vi "GetBounds 1.vi"(0 "XRef":T5, 1 "State In":T4) -> (14 "Bounds":T2, 15 "Fatal Error Out":T1)   [LabVIEW 2012, in "VireoFunctionNode.xnode"]
uses:
  VireoFunctionNode.xnode
  <vilib>/XNodeSupport/XNodeXNodeRef.ctl
  State 1.ctl
  <vilib>/XNodeSupport/XNodeBounds.ctl
  <vilib>/XNodeSupport/XNodeInt.ctl
  <vilib>/XNodeSupport/XNodeErrorCluster.ctl
  <vilib>/XNodeSupport/NI_XNodeSupport.lvlib
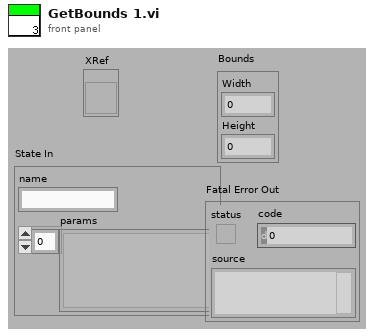
[diagram p1: front panel]
types:
  T1 = typedef "NI_XNodeSupport.lvlib/XNodeErrorCluster.ctl" = errorcluster
  T2 = typedef "NI_XNodeSupport.lvlib/XNodeBounds.ctl" = cluster{"Width":T3, "Height":T3}
  T3 = typedef "NI_XNodeSupport.lvlib/XNodeInt.ctl" = i32
  T4 = typedef "VireoFunctionNode.xnode/State 1.ctl" = cluster{"name":string, "params":variant[]}
  T5 = typedef "NI_XNodeSupport.lvlib/XNodeXNodeRef.ctl" = refnum<vi>
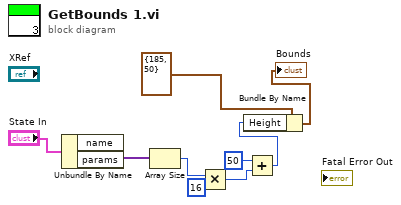
[diagram p0: block diagram]
diagram:
  n1 = Unbundle By Name("State In") -> ("params"=w8:variant[])  [unwired: 1 out]
  n2 = Array Size(array=w8) -> (size(s)=w7:i32)
  n3 = Multiply(x=w7, y=16) -> (x*y=w5:i32)
  n4 = Add(x=50, y=w5) -> (x+y=w3:i32)
  n5 = Bundle By Name(cluster=T2 {"Width"=185, "Height"=50} ("Bounds"), "Height"=w3) -> (→"Bounds":T2)
